vi "pose.vi"(0 "Pose":T1={"X"=0.1, "Y"=0.1, "Z"=0.1, "roll"=0.1, "pitch"=0.1, "yaw"=0.1}) -> (4 "sdf out":string)   [LabVIEW 2010]
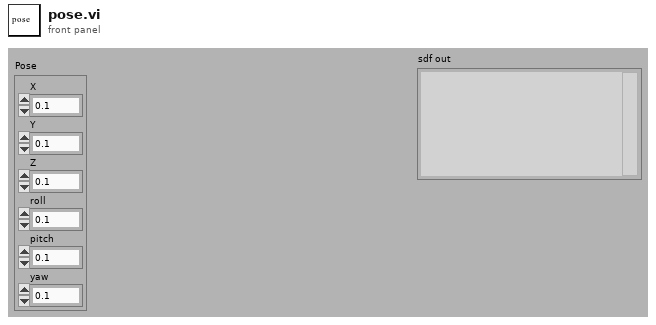
[diagram p1: front panel]
types:
  T1 = cluster{"X":sgl, "Y":sgl, "Z":sgl, "roll":sgl, "pitch":sgl, "yaw":sgl}
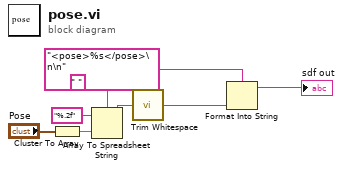
[diagram p0: block diagram]
diagram:
  n1 = Cluster To Array(cluster="Pose") -> (array=w7:sgl[])
  n2 = Array To Spreadsheet String(delimiter (Tab)=" ", array=w7, 3:"%.2f" ("format string")) -> (spreadsheet string=w4:string)
  n3 = call <vilib>:"Trim Whitespace.vi"("string"=w4) -> ("trimmed string"=w1:string)  [unwired: 1 in]
  n4 = Format Into String(format string="<pose>%s</pose>\n\n", w1) -> (resulting string=→"sdf out":string)  [unwired: 2 in, 1 out]
